vi "Unregister.vi"(8 "error in":errorcluster, 11 "epoll in":refnum<class "epoll.lvclass">) -> (0 "error out":errorcluster, 3 "epoll out":refnum<class "epoll.lvclass">)   [LabVIEW 2019, in "PCANBasic.lvlib" / "epoll.lvclass"]
uses:
  epoll.lvclass
  epoll.lvclass/epoll.ctl
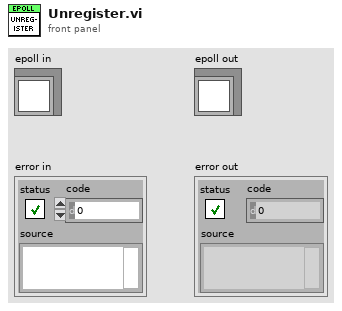
[diagram p1: front panel]
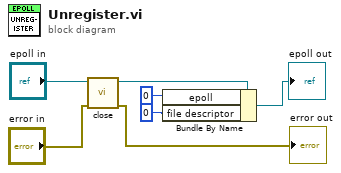
[diagram p0: block diagram]
diagram:
  n1 = call "close.vi"("error in"="error in", "epoll in"="epoll in") -> ("error out"=→"error out":errorcluster, "epoll out"=w6:refnum<class "epoll.lvclass">)  [unwired: 8 in]
  n2 = Bundle By Name(cluster=w6, "epoll"=0, "file descriptor"=0) -> (→"epoll out":refnum<class "epoll.lvclass">)
